vi "S2DS_Find Port Number (SubVI).vi"(11 "String":string) -> (2 "Port No (String)":string, 3 "Numeric":i32)   [LabVIEW 2025]
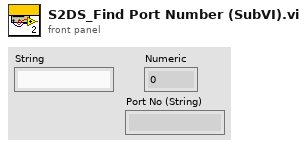
[diagram p1: front panel]
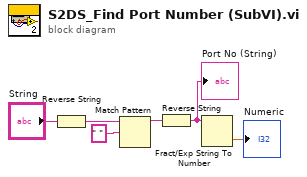
[diagram p0: block diagram]
diagram:
  n1 = Reverse String(1:"String") -> (0:w1:string)
  n2 = Match Pattern(string=w1, regular expression=" ") -> (before substring=w3:string)  [unwired: 1 in, 3 out]
  n3 = Reverse String(1:w3) -> (0:w5:string)
  "Port No (String)" <- w5
  n4 = Fract/Exp String To Number(string=w5) -> (number=→"Numeric":dbl)  [unwired: 3 in, 1 out]
